vi "VelocityVoltage SetControl.vi"(0 "DeviceReference":T1, 1 "StopSendingOtherRequests":bool=TRUE, 2 "Velocity":dbl, 3 "Acceleration":dbl, 4 "EnableFOC":bool=TRUE, 5 "FeedForward":dbl, 6 "Slot":i32, 7 "error in":errorcluster, 8 "OverrideBrakeDurNeutral":bool, 9 "LimitForwardMotion":bool, 10 "LimitReverseMotion":bool, 18 "Update Frequency (Hz)":dbl=100.0) -> (20 "DeviceReference Out":T1, 27 "error out":errorcluster)   [LabVIEW 2023]
doc: "Request PID to target velocity with voltage feedforward.\nThis control mode will set the motor's velocity setpoint to the velocity specified by the user. In addition, it will apply an additional voltage as an arbitrary feedforward value."
uses:
  <vilib>/Rock Robotics/WPI/ThirdParty/Phoenix6/DeviceReference.ctl
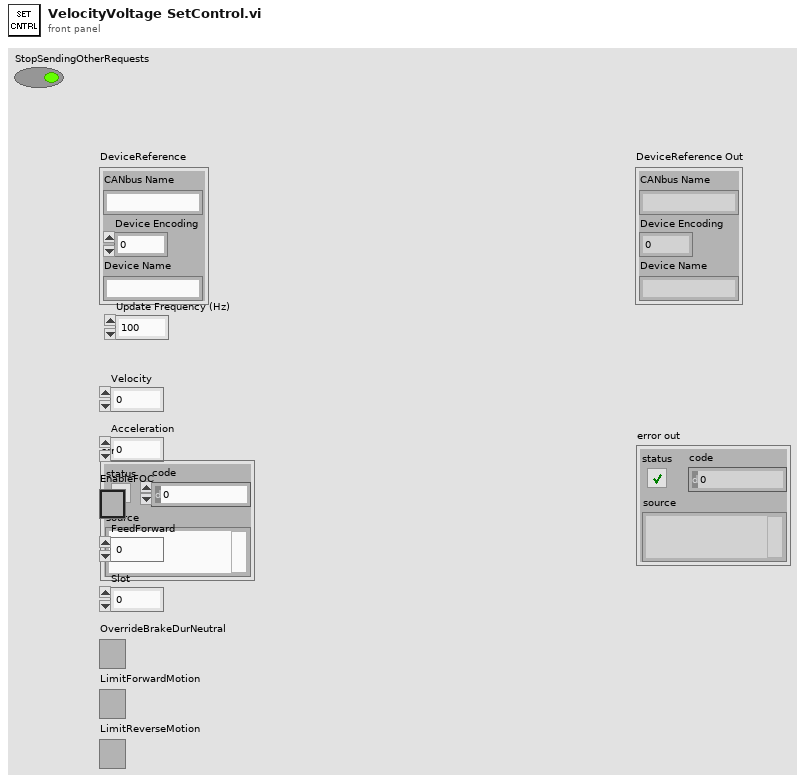
[diagram p1: front panel]
types:
  T1 = typedef "DeviceReference.ctl" = cluster{"CANbus Name":string, "Device Encoding":u32, "Device Name":string}
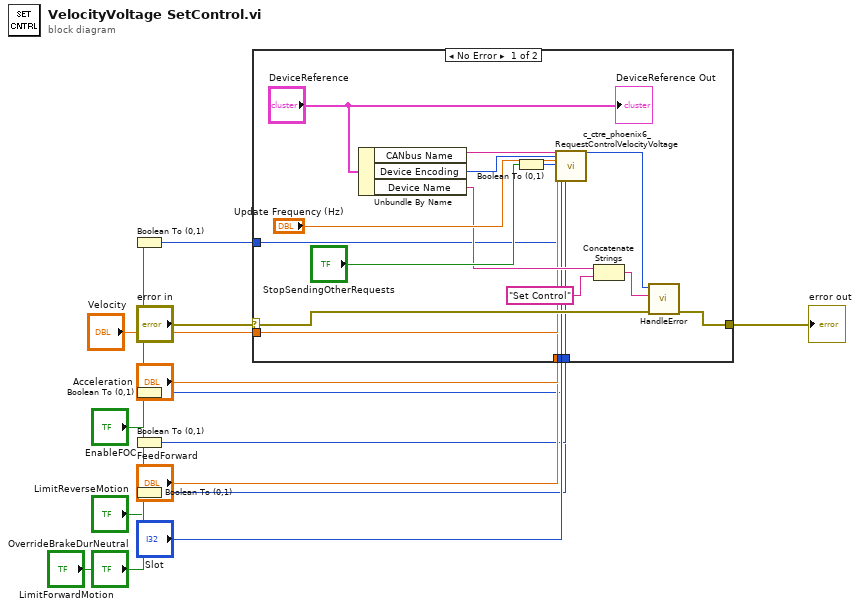
[diagram p0: block diagram]
diagram:
  n1 = Boolean To (0,1)(Boolean="EnableFOC") -> (0, 1=w9:i16)
  n2 = Boolean To (0,1)(Boolean="OverrideBrakeDurNeutral") -> (0, 1=w5:i16)
  n3 = Boolean To (0,1)(Boolean="LimitForwardMotion") -> (0, 1=w3:i16)
  n4 = Boolean To (0,1)(Boolean="LimitReverseMotion") -> (0, 1=w1:i16)
  n5 = case shown="No Error" "error in" {
    selector: "error in" -> [w27 w35]
    tunnel: [w26 w35] -> w13
    tunnel: "Velocity" -> [w22 _]
    tunnel: "Acceleration" -> [w21 _]
    tunnel: w9 -> [w20 _]
    tunnel: "FeedForward" -> [w19 _]
    tunnel: "Slot" -> [w18 _]
    tunnel: w5 -> [w17 _]
    tunnel: w3 -> [w16 _]
    tunnel: w1 -> [w15 _]
    frame No Error {
      n6 = Unbundle By Name("DeviceReference") -> ("CANbus Name"=w33:string, "Device Encoding"=w32:u32, "Device Name"=w25:string)
      n7 = Boolean To (0,1)(Boolean="StopSendingOtherRequests") -> (0, 1=w29:i16)
      n8 = call <vilib>:"c_ctre_phoenix6_RequestControlVelocityVoltage.vi"("String 2"=w33, "Numeric 2"=w32, "Numeric 3"="Update Frequency (Hz)", "Numeric 4"=w29, "Numeric 5"=w22, "Numeric 6"=w21, "Numeric 7"=w20, "Numeric 8"=w19, "Numeric 9"=w18, "Numeric 10"=w17, "Numeric 11"=w16, "Numeric 12"=w15) -> ("Numeric"=w28:i32)  [unwired: 14 in, 1 out]
      n9 = Concatenate Strings(w25, "Set Control" ("origin")) -> (w23:string)
      n10 = call <vilib>:"HandleError.vi"("error in"=w27, "origin"=w23, "Status"=w28) -> ("error out"=w26:errorcluster)  [unwired: 8 in]
      "DeviceReference Out" <- "DeviceReference"
    }
    frame Error {
    }
  }
  "error out" <- w13
